vi "RobotGlobal.vi"() -> ()   [LabVIEW 2018]
uses:
  TypeDefs/RobotObjects.ctl
  Classes/Drive/Drive.lvclass
  Classes/Pnematics control/Pneumatics.lvclass
  Classes/Vision/Vision.lvclass
  Classes/Joysticks/Joysticks.lvclass
  Classes/Elevator/Elevator.lvclass
  Classes/Hatch/Hatch.lvclass
  Classes/Cargo/Cargo.lvclass
panel:
  in  "CodeConfigFile":path
  in  "RobotData":T1
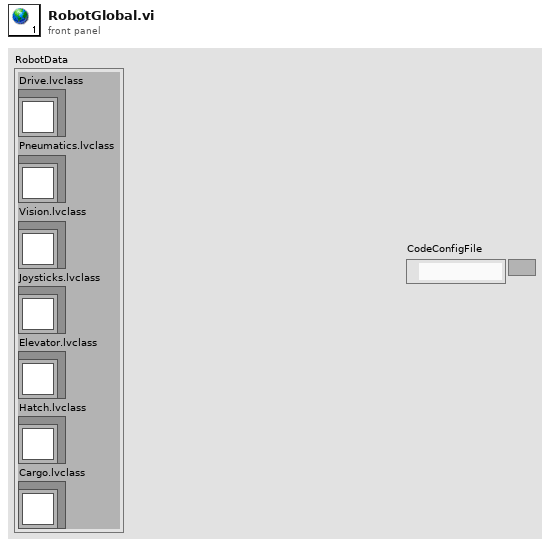
[diagram p1: front panel]
types:
  T1 = typedef "RobotObjects.ctl" = cluster{"Drive.lvclass":refnum<class "Drive.lvclass">, "Pneumatics.lvclass":refnum<class "Pneumatics.lvclass">, "Vision.lvclass":refnum<class "Vision.lvclass">, "Joysticks.lvclass":refnum<class "Joysticks.lvclass">, "Elevator.lvclass":refnum<class "Elevator.lvclass">, "Hatch.lvclass":refnum<class "Hatch.lvclass">, "Cargo.lvclass":refnum<class "Cargo.lvclass">}
diagram:
